vi "Can_RecData.vi"(6 "timeout":u32=3000, 7 "mode":enum16{"Init", "Rec"}(ring)=enum."Rec", 8 "error in (no error)":errorcluster, 9 "Interface:Baud Rate":u32=250000, 10 "cluster (:memory:)":refnum<k21>=":memory:", 11 "interface":refnum<k21>) -> (0 "error out":errorcluster, 2 "data":T1[](array[typedef]) {"payload" format="%x"; "timestamp" format="%<%.7X\n%x>T"; "type" items=["CAN Data"=0, "CAN Remote"=1, "CAN Bus Error"=2, "CAN 2.0 Data"=8, "CAN FD Data"=16, "CAN FD+BRS Data"=24, "J1939 Data"=192, "Delay"=224, "Log Trigger"=225, "Start Trigger"=226]; "identifier" format="%x"}, 4 "RespGood？":bool)   [LabVIEW 2015]
uses:
  <vilib>/xnet/xnet.llb/XNET Frame CAN.ctl
  <vilib>/xnet/xnet.llb/XNET Frame Type CAN.ctl
  <vilib>/xnet/xnet.llb/XNET Create Session (Frame Input Stream).vi
  <vilib>/xnet/xnet.llb/XNET Read (Frame CAN).vi
  <resource>/objmgr/xnet.rc
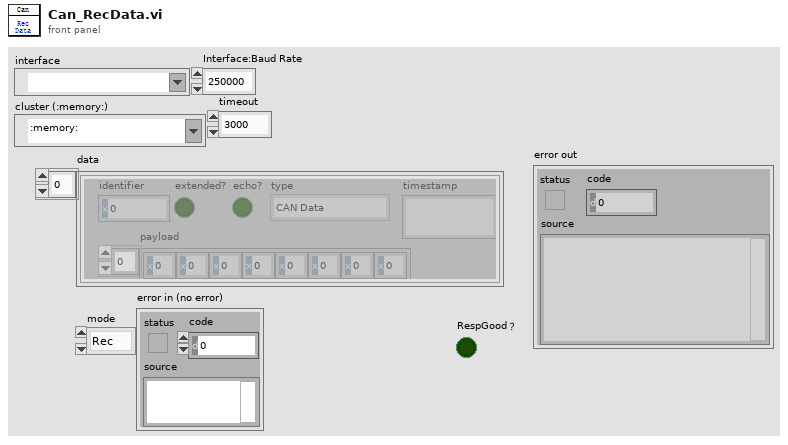
[diagram p1: front panel]
types:
  T1 = typedef "XNET Frame CAN.ctl" = cluster{"timestamp":timestamp, "payload":u8[], "identifier":u32, "type":T2, "extended?":bool, "echo?":bool}
  T2 = typedef "XNET Frame Type CAN.ctl" = u8
  T3 = cluster{"session":refnum<k21>, "error":errorcluster}
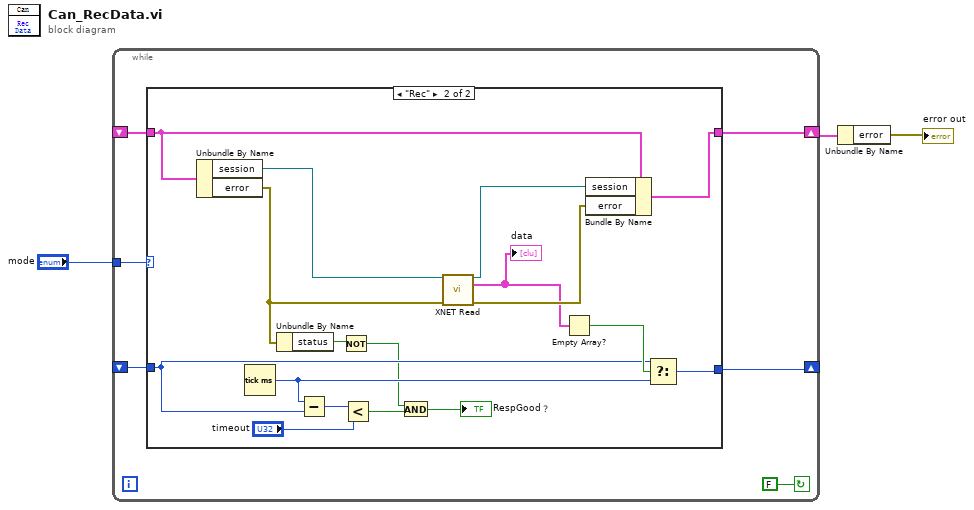
[diagram p0: block diagram]
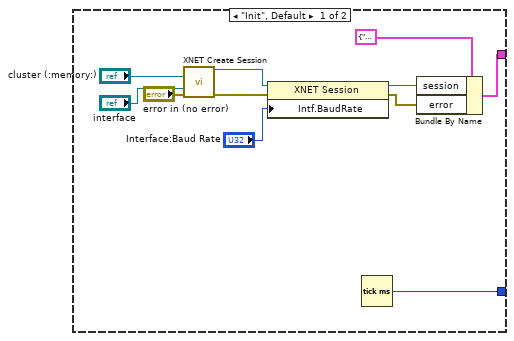
[diagram p2: hidden frame]
diagram:
  n1 = while {
    tunnel: "mode" -> [w8]
    shift-right: [w6] -> w2
    shift-left: _ -> [w7]
    shift-right: [w5] -> _
    shift-left: _ -> [w4]
    stop <- FALSE continue-if-true
    n2 = case shown="\"Rec\"" w8 {
      tunnel: w7 -> [_ w36]
      tunnel: [w13 w33] -> w6
      tunnel: [w10 w30] -> w5
      tunnel: w4 -> [_ w28]
      frame "Init", Default {
        n3 = call-poly <vilib>:"XNET Create Session.vi"("cluster (:memory:)"="cluster (:memory:)", "interface"="interface", "error in (no error)"="error in (no error)") -> ("session out"=w18:refnum<k21>, "error out"=w19:errorcluster)  [unwired: 11 out]
        n4 = property class="XNET Session"(reference=w18, error in=w19, "Intf.BaudRate"="Interface:Baud Rate") -> (reference out=w15:refnum<k21>, error out=w14:errorcluster)
        n5 = Tick Count (ms)() -> (millisecond timer value=w10:u32)
        n6 = Bundle By Name(cluster=T3 {"session"="", "error"={"status"=FALSE, "code"=0, "source"=""}}, "session"=w15, "error"=w14) -> (w13:T3)
      }
      frame "Rec" {
        n7 = Unbundle By Name(w36) -> ("session"=w37:refnum<k21>, "error"=w23:errorcluster)
        n8 = Tick Count (ms)() -> (millisecond timer value=w27:u32)
        n9 = Unbundle By Name(w23) -> ("status"=w22:bool)
        n10 = Subtract(x=w27, y=w28) -> (x-y=w31:u32)
        n11 = Not(x=w22) -> (.not. x?=w21:bool)
        n12 = Less?(x=w31, y="timeout") -> (x < y?=w25:bool)
        n13 = And(x=w21, y=w25) -> (x .and. y?=→"RespGood？":bool)
        n14 = call-poly <vilib>:"XNET Read.vi"("session in"=w37, "error in (no error)"=w23) -> ("session out"=w35:refnum<k21>, "data"=w32:T1[], "error out"=w34:errorcluster)  [unwired: 11 out]
        "data" <- w32
        n15 = Empty Array?(array=w32) -> (empty?=w29:bool)
        n16 = Bundle By Name(cluster=w36, "session"=w35, "error"=w34) -> (w33:T3)
        n17 = Select(t=w28, s=w29, f=w27) -> (s? t:f=w30:u32)
      }
    }
  }
  n18 = Unbundle By Name(w2) -> ("error"=→"error out":errorcluster)
